vi "waitForFPactivityExample.vi"() -> ()   [LabVIEW 2021]
panel:
  out "Numeric":i32
  in  "Wait?":bool
  out "current time":timestamp
  out "sum":dbl
  in  "Vertical Pointer Slide 2":dbl(slide) scale=0.0..10.0
  in  "Vertical Pointer Slide":dbl(slide) scale=0.0..10.0
  in  "Stop":bool
  # "Press this, and notice the current time doesn't continually increment- only if FP changed ->"
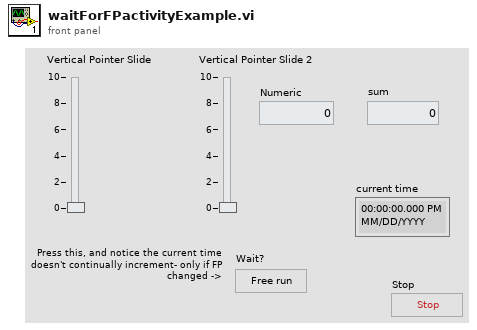
[diagram p1: front panel]
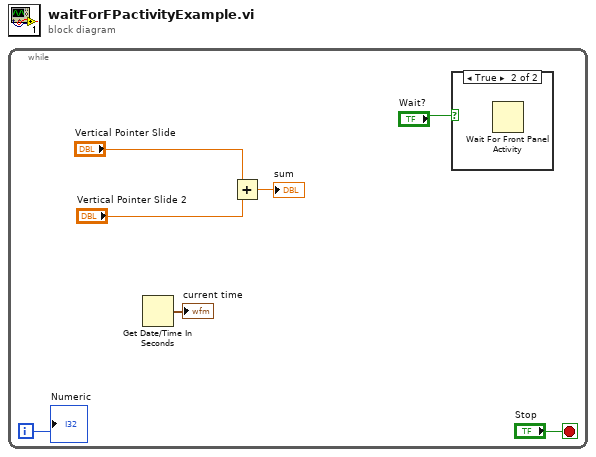
[diagram p0: block diagram]
diagram:
  n1 = while {
    i -> [w1]
    stop <- "Stop" stop-if-true
    n2 = Get Date/Time In Seconds() -> (seconds since 1Jan1904=→"current time":timestamp)
    n3 = Add(x="Vertical Pointer Slide", y="Vertical Pointer Slide 2") -> (x+y=→"sum":dbl)
    n4 = case shown="True" "Wait?" {
      frame False {
      }
      frame True {
        n5 = Wait For Front Panel Activity() -> ()  [unwired: 3 in, 1 out]
      }
    }
    "Numeric" <- w1
  }
